vi "食物生成.vi"(10 "上限":dbl, 11 "数组输入":cluster{"x":dbl, "y":dbl}[](array[cluster])) -> (3 "输出点":cluster{"x":dbl, "y":dbl})   [LabVIEW 2012]
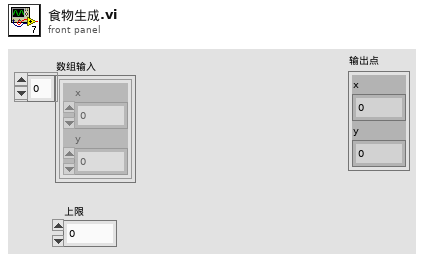
[diagram p1: front panel]
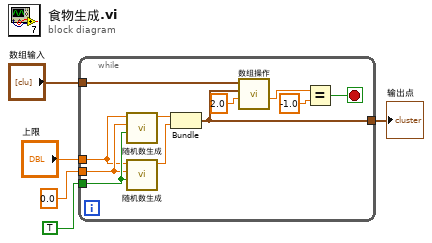
[diagram p0: block diagram]
diagram:
  n1 = while {
    tunnel: TRUE ("整数/浮点") -> [w16]
    tunnel: 0.0 ("下限") -> [w15]
    tunnel: "上限" -> [w14]
    tunnel: "数组输入" -> [w10]
    tunnel: [w6] -> w1
    stop <- w7 stop-if-true
    n2 = call "随机数生成.vi"("整数/浮点"=w16, "下限"=w15, "上限"=w14) -> ("输出"=w13:dbl)  [unwired: 8 in]
    n3 = call "随机数生成.vi"("整数/浮点"=w16, "下限"=w15, "上限"=w14) -> ("输出"=w12:dbl)  [unwired: 8 in]
    n4 = Bundle("输出"=w13, "输出"=w12) -> (w6:cluster{"输出":dbl, "输出":dbl})  [unwired: 1 in]
    n5 = call "数组操作.vi"("操作码"=2.0, "输入点"=w6, "数组输入"=w10) -> ("索引"=w9:dbl)  [unwired: 6 in, 2 out]
    n6 = Equal?(x=w9, y=-1.0) -> (x = y?=w7:bool)
  }
  "输出点" <- w1
